vi "Active Power-Spectrum Method.vi"() -> ()   [LabVIEW 2014]
uses:
  <vilib>/DAQmx/create/channels.llb/DAQmx Create Channel (AI-Voltage-Basic).vi
  <vilib>/DAQmx/configure/timing.llb/DAQmx Timing (Sample Clock).vi
  <vilib>/DAQmx/read.llb/DAQmx Read (Analog 1D DBL 1Chan NSamp).vi
panel:
  in  "fig-index":i32
  out "size(s)":i32[](array[numeric])
  out "Power Spectrum (V^2 rms) (V^2)":dbl[][](array[numeric])
  out "physical channels":tag
  out "all cycles PSD":dbl[][](array[numeric])
  out "stiffness from diffusion coeff.(pN/nm)":dbl
  in  "Temp (C)":dbl
  out "stiffness from friction coeff.(pN/nm)":dbl
  out "Diffusion coefficient, D (V^2/s)":dbl
  out "a1":dbl
  in  "bead height (um)":dbl=1.0
  in  "bead radius (um)":dbl=0.515
  out "Beta (V/um)":dbl
  out "fResponse (Hz)":dbl
  out "Wex":dbl
  out "Wth":dbl
  out "fc":dbl
  out "best fit parameters\n(XX,fc)":dbl[](array[numeric])
  in  "Freq End Cut":dbl
  in  "Freq Strat Cut":dbl
  out "Frequency (Hz)\n0,df, 2df,...(n/2-1)Fs":dbl[](array[numeric])
  out "Avg. PSD":dbl[](array[numeric])
  out "Avg. completed":i32
  in  "Tab Control":enum32{"Page 1", "Page 3", "Page 2"}(tab)
  out "XY Graph":T1(graph)
  out "XY Graph 3":T2(graph)
  out "XY Graph 2":T3(graph)
  in  "Cycles to average":i32=30
  in  "Sampling Rate (Hz)":dbl=32000.0 format="%0.2f"
  out "Need time (s)":dbl format="%.5f"
  in  "Amplitude, A (nm)":dbl=200.0
  in  "f_drive (Hz)":dbl=30.0
  in  "Axis":enum16{"x", "y", "z"}(ring)
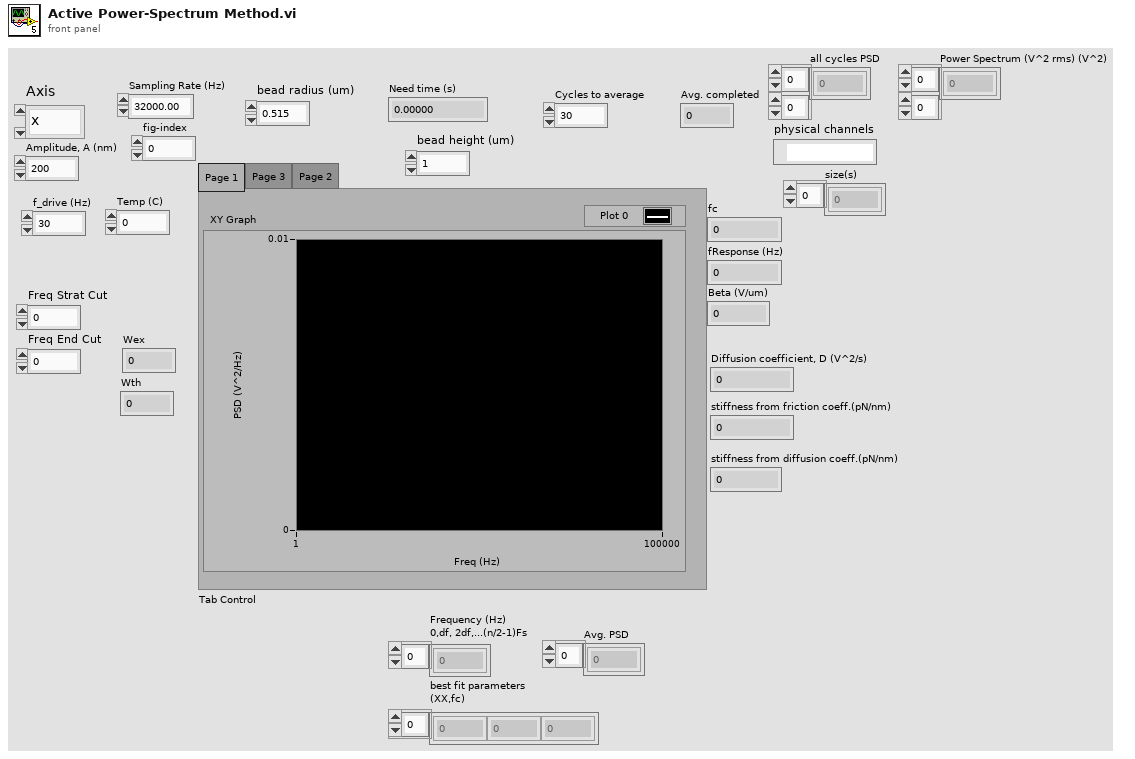
[diagram p1: front panel]
types:
  T1 = cluster{"Frequency (Hz)\n0,df, 2df,...(n/2-1)Fs":dbl[], dbl[]}
  T2 = cluster{"Frequency (Hz)\n0,df, 2df,...(n/2-1)Fs":dbl[], "Power Spectrum (V^2 rms) (V^2)":dbl[]}
  T3 = cluster{"Frequency (Hz)\n0,df, 2df,...(n/2-1)Fs":dbl[], dbl[]}[]
  T4 = cluster{"Freq Cut":dbl[], "best nonlinear fit PSD":dbl[]}
  T5 = cluster{"Frequency (Hz)\n0,df, 2df,...(n/2-1)Fs":dbl[], "best nonlinear fit PSD":dbl[]}[]
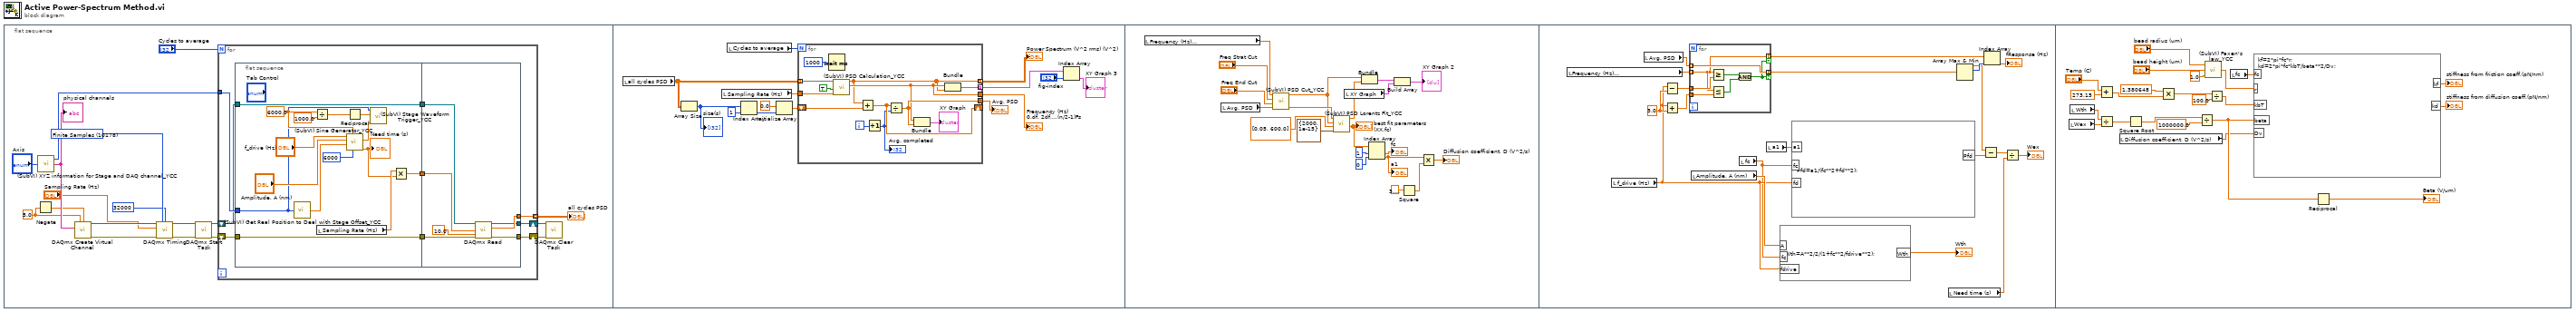
[diagram p0: block diagram]
diagram:
  n1 = flat-sequence {
    frame #0 {
      w7 = 10178 items=["Finite Samples"=10178, "Continuous Samples"=10123, "Hardware Timed Single Point"=12522] ("sample mode")
      w13 = 5.0 ("maximum value")
      n2 = Negate(x=w13) -> (-x=w12:dbl)
      n3 = call "(SubVI) XYZ information for Stage and DAQ channel_YCC.vi"("Axis  (Enum)"="Axis") -> ("physical channels"=w14:tag, "Axis"=w17:i32)  [unwired: 3 in]
      "physical channels" <- w14
      n4 = call-poly <vilib>:"DAQmx Create Virtual Channel.vi"("maximum value"=w13, "minimum value"=w12, "physical channels"=w14) -> ("task out"=w9:refnum<k21>, "error out"=w8:errorcluster)  [unwired: 11 in]
      n5 = call-poly <vilib>:"DAQmx Timing.vi"("task/channels in"=w9, "sample mode"=w7, "samples per channel"=32000, "rate"="Sampling Rate (Hz)", "error in"=w8) -> ("task out"=w11:refnum<k21>, "error out"=w10:errorcluster)  [unwired: 2 in, 7 out]
      n6 = call <vilib>:"DAQmx Start Task.vi"("task/channels in"=w11, "error in"=w10) -> ("task out"=w4:refnum<k21>, "error out"=w3:errorcluster)  [unwired: 12 out]
      n7 = for {
        N: "Cycles to average" -> [_]
        tunnel: w17 -> [w26]
        tunnel: [w25] -> w16 mode=indexing
        shift-right: [w24] -> w2
        shift-left: w4 -> [w21]
        shift-right: [w23] -> w1
        shift-left: w3 -> [w19]
        n8 = flat-sequence {
          tunnel: w26 -> [w33]
          tunnel: [w31] -> w27
          tunnel: [w29] -> w22
          tunnel: w21 -> [w29]
          tunnel: [w28] -> w20
          tunnel: w19 -> [w28]
          tunnel: [w49] -> w25
          tunnel: [w48] -> w24
          tunnel: [w47] -> w23
          tunnel: w20 -> [w43]
          tunnel: w22 -> [w44]
          tunnel: w27 -> [w46]
          frame #0 {
            w39 = 6000.0 ("fs (Hz)")
            n9 = call "(SubVI) Get Real Position to Deal with Stage Offset_YCC.vi"("Axis"=w33) -> ("Real Current Commanded position (um)"=w42:dbl)  [unwired: 3 in, 1 out]
            n10 = Divide(x=w39, y=1000.0) -> (x/y=w37:dbl)
            n11 = local read "Sampling Rate (Hz)"() -> (w32:dbl)
            n12 = call "(SubVI) Sine Generator_YCC.vi"("Points to be generated"=6000, "fs (Hz)"=w39, "initial position (um)"=w42, "Amplitude, A (nm)"="Amplitude, A (nm)", "f_drive (Hz)"="f_drive (Hz)") -> ("Total Need time (s)"=w30:dbl, "Position Array (um)"=w35:dbl[])  [unwired: 1 in, 2 out]
            "Need time (s)" <- w30
            n13 = Reciprocal(x=w37) -> (1/x=w36:dbl)
            n14 = call "(SubVI) Stage Waveform Trigger_YCC.vi"("Position Array (um)"=w35, "milliseconds to wait"=w36, "axis"=w33) -> ()  [unwired: 5 in]
            n15 = Multiply(x=w32, y=w30) -> (x*y=w31:dbl)
          }
          frame #1 {
            n16 = call-poly <vilib>:"DAQmx Read.vi"("task/channels in"=w44, "number of samples per channel"=w46, "timeout"=10.0, "error in"=w43) -> ("task out"=w48:refnum<k21>, "data"=w49:dbl[], "error out"=w47:errorcluster)  [unwired: 9 in]
          }
        }
      }
      "all cycles PSD" <- w16
      n17 = call <vilib>:"DAQmx Clear Task.vi"("task in"=w2, "error in"=w1) -> ()  [unwired: 13 in, 1 out]
    }
    frame #1 {
      n18 = local read "all cycles PSD"() -> (w55:dbl[][])
      n19 = Array Size(array=w55) -> (size(s)=w61:i32[])
      "size(s)" <- w61
      n20 = local read "Sampling Rate (Hz)"() -> (w63:dbl)
      n21 = local read "Cycles to average"() -> (w53:i32)
      n22 = Index Array(array=w61, index=1) -> (element=w59:i32)
      n23 = Initialize Array(0.0 ("element"), w59) -> (w58:dbl[])
      n24 = for {
        N: w53 -> [_]
        tunnel: w55 -> [w76] mode=indexing
        tunnel: w63 -> [w74]
        shift-right: [w71] -> _
        shift-left: w58 -> [w73]
        tunnel: [w66] -> w57
        tunnel: [w69] -> w56
        tunnel: [w65] -> w54 mode=indexing
        tunnel: [w64] -> w52 mode=indexing
        i -> [w72]
        n25 = Wait (ms)(milliseconds to wait=u32 1000) -> ()  [unwired: 1 out]
        n26 = call "(SubVI) PSD Calculation_YCC.vi"("sampling frequency (Hz)"=w74, "T=NI made PSD\nF=YCC made PSD"=TRUE ("T=NI made PSD\nF=YCC made PSD"), "QPD data"=w76) -> ("Frequency (Hz)\n0,df, 2df,...(n/2-1)Fs"=w66:dbl[], "Power Spectrum (V^2 rms) (V^2)"=w65:dbl[])  [unwired: 3 in]
        n27 = Add(x=w65, y=w73) -> (x+y=w71:dbl[])
        n28 = Increment(x=w72) -> (x+1=w70:i32)
        "Avg. completed" <- w70
        n29 = Divide(x=w71, y=w70) -> (x/y=w69:dbl[])
        n30 = Bundle("Frequency (Hz)\n0,df, 2df,...(n/2-1)Fs"=w66, w69) -> (→"XY Graph":T1)  [unwired: 1 in]
        n31 = Bundle("Frequency (Hz)\n0,df, 2df,...(n/2-1)Fs"=w66, "Power Spectrum (V^2 rms) (V^2)"=w65) -> (w64:T2)  [unwired: 1 in]
      }
      "Avg. PSD" <- w56
      "Frequency (Hz)\n0,df, 2df,...(n/2-1)Fs" <- w57
      "Power Spectrum (V^2 rms) (V^2)" <- w54
      n32 = Index Array(array=w52, index="fig-index") -> (element=→"XY Graph 3":T2)
    }
    frame #2 {
      n33 = local read "Frequency (Hz)\n0,df, 2df,...(n/2-1)Fs"() -> (w79:dbl[])
      n34 = local read "Avg. PSD"() -> (w78:dbl[])
      n35 = call "(SubVI) PSD Cut_YCC.vi"("PSD"=w78, "Freq End Cut"="Freq End Cut", "Freq Strat Cut"="Freq Strat Cut", "Frequency (Hz)"=w79) -> ("PSD Cut"=w94:dbl[], "Freq Cut"=w91:dbl[])  [unwired: 2 in]
      n36 = call "(SubVI) PSD Lorentz Fit_YCC.vi"("termination"=cluster{"max iteration":i32, "tolerance":dbl} {"max iteration"=2000, "tolerance"=1e-15}, "initial parameters"=dbl[] [0.05, 600.0], "Frequency (Hz)"=w91, "PSD (Vrms^2)"=w94) -> ("best fit parameters"=w87:dbl[], "best nonlinear fit PSD"=w90:dbl[])  [unwired: 2 in]
      "best fit parameters\n(XX,fc)" <- w87
      n37 = local read "XY Graph"() -> (w88:T1)
      n38 = Bundle("Freq Cut"=w91, "best nonlinear fit PSD"=w90) -> (w89:T4)  [unwired: 1 in]
      n39 = Index Array(array=w87, index #1=1 ("index"), index #2=0 ("index")) -> (element #1=→"fc":dbl, element #2=w81:dbl)
      "a1" <- w81
      n40 = Build Array(w89, w88) -> (→"XY Graph 2":T5)
      n41 = Square(x=3.141592653589793) -> (x^2=w82:dbl)
      n42 = Multiply(x=w81, y=w82) -> (x*y=→"Diffusion coefficient, D (V^2/s)":dbl)
    }
    frame #3 {
      w111 = 3.0 ("y")
      n43 = local read "Frequency (Hz)\n0,df, 2df,...(n/2-1)Fs"() -> (w112:dbl[])
      n44 = local read "f_drive (Hz)"() -> (w104:dbl)
      n45 = local read "Avg. PSD"() -> (w113:dbl[])
      n46 = Subtract(x=w104, y=w111) -> (x-y=w110:dbl)
      n47 = Add(x=w104, y=w111) -> (x+y=w109:dbl)
      n48 = for {
        tunnel: [w122] -> w108 mode=indexing if=w116
        tunnel: w113 -> [w122] mode=indexing
        tunnel: [w120] -> w107 mode=indexing if=w116
        tunnel: w112 -> [w120] mode=indexing
        tunnel: w110 -> [w121]
        tunnel: w109 -> [w119]
        n49 = Greater Or Equal?(x=w120, y=w121) -> (x >= y?=w118:bool)
        n50 = Less Or Equal?(x=w120, y=w119) -> (x <= y?=w117:bool)
        n51 = And(x=w118, y=w117) -> (x .and. y?=w116:bool)
      }
      n52 = local read "Amplitude, A (nm)"() -> (w115:dbl)
      n53 = local read "fc"() -> (w97:dbl)
      n54 = local read "a1"() -> (w103:dbl)
      n55 = formula code="Wth=A**2/2/(1+fc**2/fdrive**2);"("A"=w115, "fc"=w97, "fdrive"=w104) -> ("Wth"=→"Wth":dbl)
      n56 = formula code="Pfd=a1/(fc**2+fd**2);"("a1"=w103, "fc"=w97, "fd"=w104) -> ("Pfd"=w101:dbl)
      n57 = local read "Need time (s)"() -> (w99:dbl)
      n58 = Array Max & Min(array=w108) -> (max value=w102:dbl, max index (indices)=w106:i32)  [unwired: 2 out]
      n59 = Subtract(x=w102, y=w101) -> (x-y=w100:dbl)
      n60 = Index Array(array=w107, index=w106) -> (element=→"fResponse (Hz)":dbl)
      n61 = Divide(x=w100, y=w99) -> (x/y=→"Wex":dbl)
    }
    frame #4 {
      n62 = local read "Wex"() -> (w143:dbl)
      n63 = local read "Wth"() -> (w144:dbl)
      n64 = Add(x="Temp (C)", y=273.15) -> (x+y=w132:dbl)
      n65 = Divide(x=w144, y=w143) -> (x/y=w142:dbl)
      n66 = local read "Diffusion coefficient, D (V^2/s)"() -> (w125:dbl)
      n67 = Square Root(x=w142) -> (sqrt(x)=w141:dbl)
      n68 = Multiply(x=1.380648, y=w132) -> (x*y=w131:dbl)
      n69 = Divide(x=w141, y=1000000.0) -> (x/y=w126:dbl)
      n70 = call "(SubVI) Faxen's law_YCC.vi"("viscosity (cP)"=1.0, "bead height (um)"="bead height (um)", "bead radius (um)"="bead radius (um)") -> ("Faxen's law of friction coefficient (N/(m/s))"=w127:dbl)  [unwired: 2 in]
      n71 = Divide(x=w131, y=100.0) -> (x/y=w129:dbl)
      n72 = local read "fc"() -> (w128:dbl)
      n73 = formula code="kf=2*pi*fc*r;\nkd=2*pi*fc*kbT/beta**2/Dv;"("fc"=w128, "r"=w127, "kbT"=w129, "beta"=w126, "Dv"=w125) -> ("kf"=→"stiffness from friction coeff.(pN/nm)":dbl, "kd"=→"stiffness from diffusion coeff.(pN/nm)":dbl)
      n74 = Reciprocal(x=w126) -> (1/x=→"Beta (V/um)":dbl)
    }
  }
